vi "STAV Write.vi"(8 "error in (no error)":errorcluster, 10 "Command":string, 11 "STAV ref in":refnum<visa-resource-name>) -> (0 "error out":errorcluster, 3 "STAV ref out":refnum<visa-resource-name>)   [LabVIEW 2021, in "STAV lib.lvlib"]
uses:
  STAV lib.lvlib
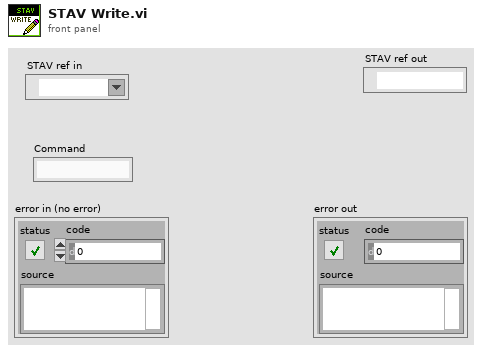
[diagram p1: front panel]
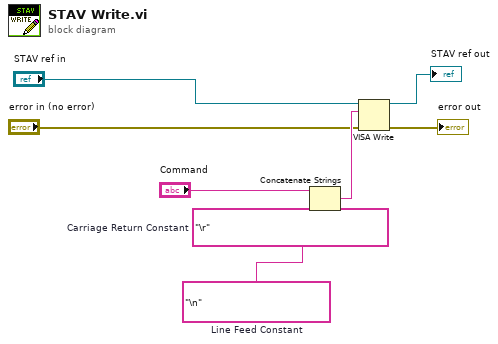
[diagram p0: block diagram]
diagram:
  w6 = "\r"  # Carriage Return Constant
  w7 = "\n"  # Line Feed Constant
  n1 = Concatenate Strings("Command", w6, w7) -> (w8:string)
  n2 = VISA Write(VISA resource name="STAV ref in", write buffer=w8, error in (no error)="error in (no error)") -> (VISA resource name out=→"STAV ref out":refnum<visa-resource-name>, error out=→"error out":errorcluster)  [unwired: 1 out]
